vi "Error Process.vi"(8 "error in (no error)":errorcluster, 11 "View Model":T1) -> (0 "error out":errorcluster)   [LabVIEW 2017]
doc: "Responsible for collecting and handling all errors"
uses:
  View Model/Controls/View Model.ctl
  Controls/Error Model.ctl
  Controls/Error Type.ctl
  View Model/Controls/Shared Model.ctl
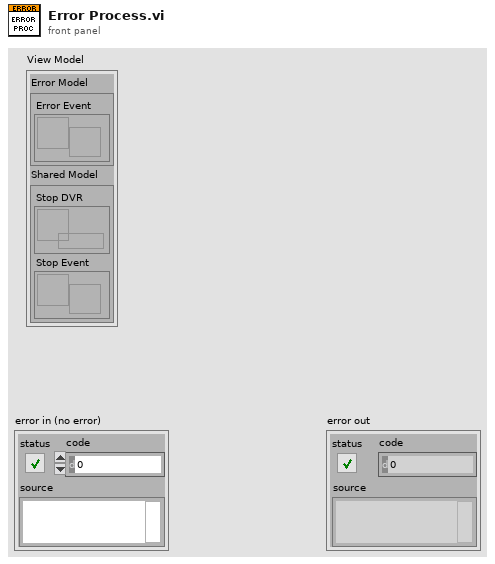
[diagram p1: front panel]
types:
  T1 = typedef "View Model.ctl" = cluster{"Error Model":T2, "Shared Model":T3}
  T2 = typedef "Error Model.ctl" = cluster{"Error Event":refnum<user-event>}
  T3 = typedef "Shared Model.ctl" = cluster{"Stop DVR":refnum<data-value>, "Stop Event":refnum<user-event>}
  T4 = typedef "Error Type.ctl" = enum16{"Console Error", "Process Step Error", "Sensor Interface IO Error"}
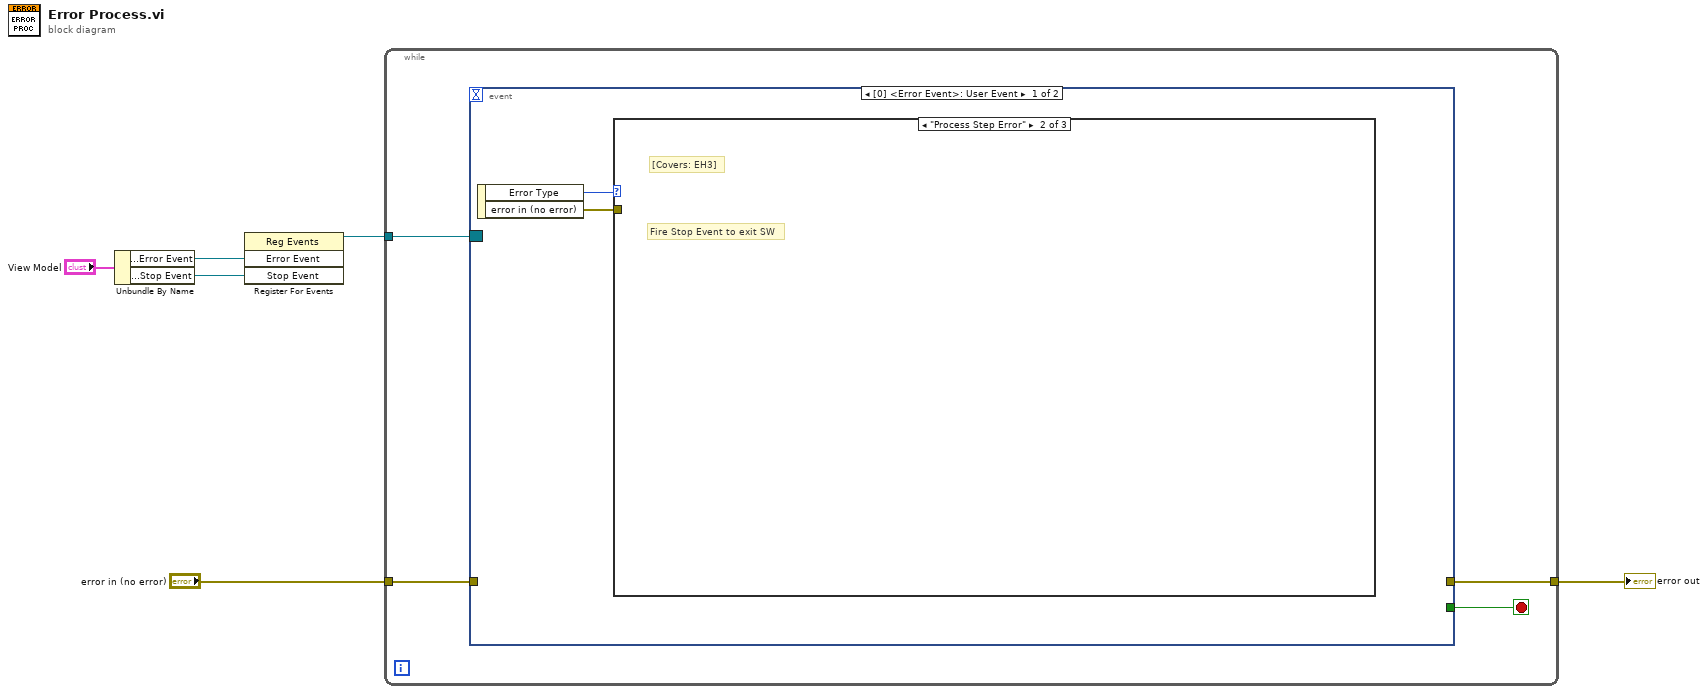
[diagram p0: block diagram]
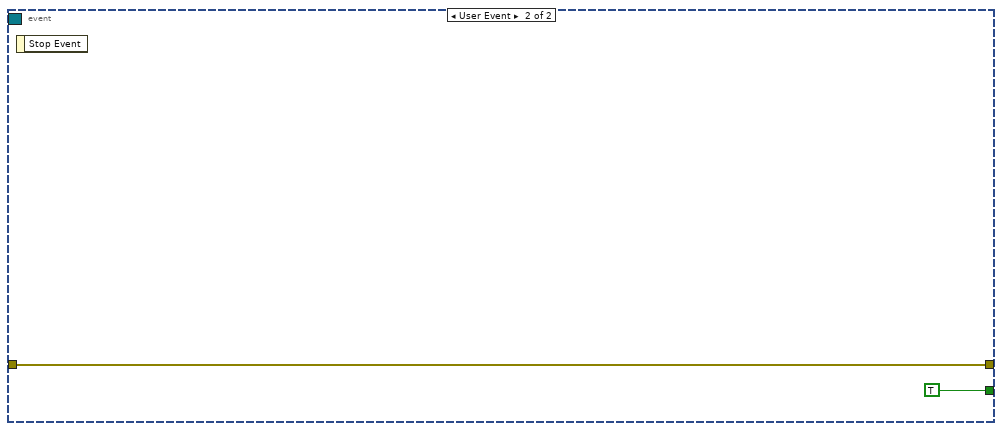
[diagram p4: hidden frame]
diagram:
  n1 = Unbundle By Name("View Model") -> ("Error Model.Error Event"=w5:refnum<user-event>, "Shared Model.Stop Event"=w3:refnum<user-event>)
  n2 = register-events(w5, w3) -> (reference out=w4:refnum<event-registration>)  [unwired: 2 in, 1 out]
  n3 = while {
    tunnel: w4 -> [w10]
    tunnel: "error in (no error)" -> [w8]
    tunnel: [w7] -> w1
    stop <- w9 stop-if-true
    n4 = event shown="[0] <Error Event>: User Event" {
      selector: w10 -> [_ _]
      dyn-events: _ -> [_ _]
      timeout: _ -> [_ _]
      tunnel: [_ TRUE] -> w9
      tunnel: w8 -> [_ w13]
      tunnel: [_ w13] -> w7
      event User Event {
        n5 = event-data() -> ("Error Type"=w12:T4, "error in (no error)"=w11:errorcluster)  [unwired: 1 in]
        n6 = case shown="\"Process Step Error\"" w12 {
          tunnel: w11 -> [_ _ _]
          frame "Console Error", Default {
            # "[Covers: EH1B2]"
            # "[Covers: EH1B1]"
            # "[Covers: EH1B]"
            # "[Covers: EH1A]"
            # "[Covers: EH1]"
            # "Console Error: Alert user.\nIf error source = Display Console View, notify user and clear error\n\nIf error source = User Console View, Allow user to choose to clear\nor continue w/error.\n- If error cleared, continue last operation.\n- If continue, process error as a \"Process Step Error\""
          }
          frame "Process Step Error" {
            # "Fire Stop Event to exit SW"
            # "[Covers: EH3]"
          }
          frame "Sensor Interface IO Error" {
            # "Fire Stop Event to exit SW"
            # "[Covers: EH2]"
          }
        }
      }
      event User Event {
        n7 = event-data() -> ()  [unwired: 1 in, 1 out]
      }
    }
  }
  "error out" <- w1
